vi "Traverse.vi"() -> ()   [LabVIEW 2011]
uses:
  Anemometry/Anemometry Sub Vis/Controls/User_Specific_mode.ctl
  Anemometry/Anemometry Sub Vis/Controls/Tunnel_Coordinates.ctl
  Anemometry/Anemometry Sub Vis/Gen Trav/Trav_mode.ctl
  <vilib>/Utility/file.llb/Write To Spreadsheet File (DBL).vi
panel:
  in  "Loop Delay (s)":u32=15
  in  "Minimum Depth into soution (mm)":dbl=1120.0
  in  "Number of Points Between Minimum and Maximum Depth":dbl=20.0
  in  "Maximum Depth into solution (mm)":dbl=1399.0
  in  "Save Location":path=path "C:/Documents and Settings/Adetola Elias/My Documents/Danial/Traverse Run Actual.xls"
  in  "Sample Size for Density Meter Reading":i32=20
  in  "Delay For Density Meter Reading (s)":u32=15
  # "Time from Traverse to Density Meter = 14 Sec"
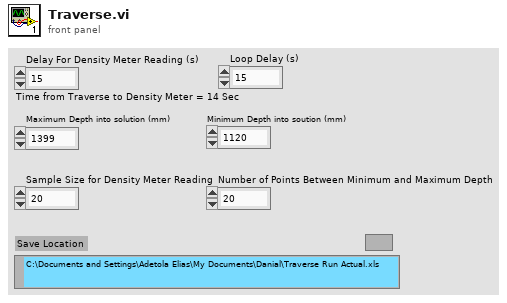
[diagram p1: front panel]
types:
  T1 = typedef "User_Specific_mode.ctl" = enum16{"Check VI only", "Run VI"}
  T2 = typedef "Tunnel_Coordinates.ctl" = enum16{"Work in Tunnel Coordinates", "Work in Model Coordinates"}
  T3 = typedef "Trav_mode.ctl" = enum16{"Move traverse", "Read traverse position", "Teach Position"}
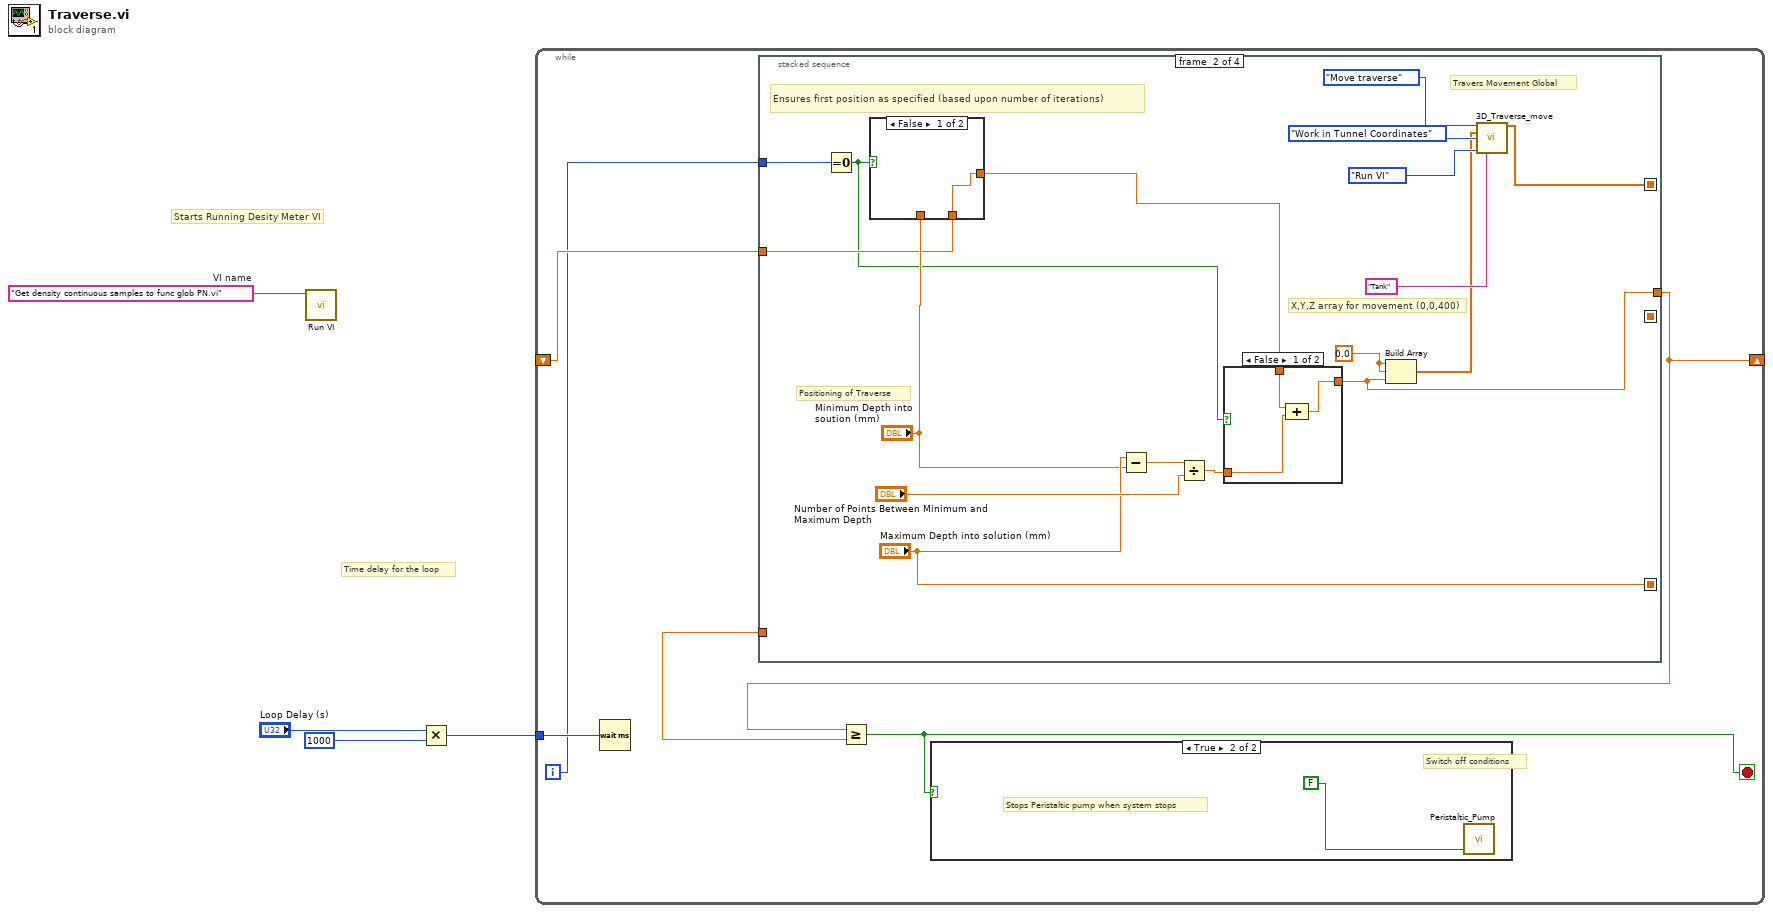
[diagram p0: block diagram]
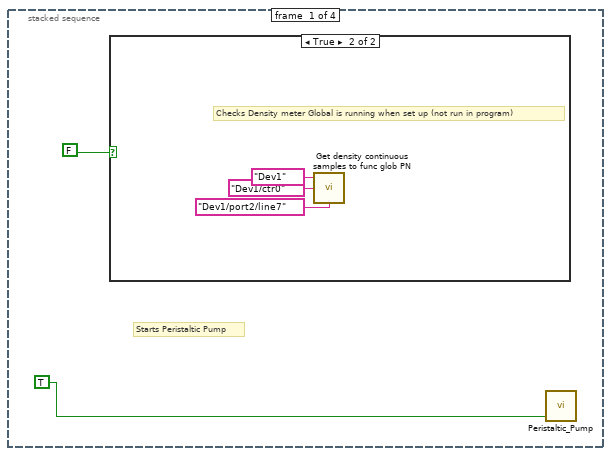
[diagram p3: hidden frame]
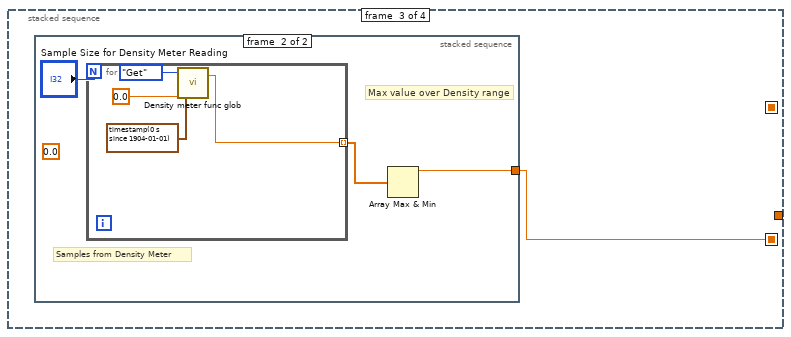
[diagram p7: hidden frame]
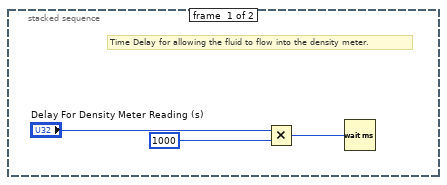
[diagram p8: hidden frame]
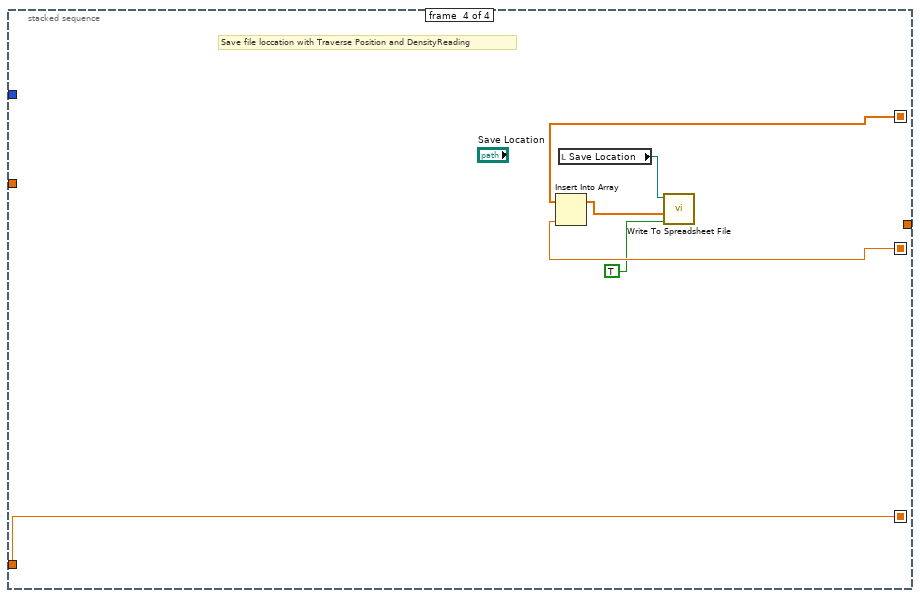
[diagram p9: hidden frame]
diagram:
  w3 = "Get density continuous samples to func glob PN.vi"  # VI name
  # "Time delay for the loop"
  # "Starts Running Desity Meter VI"
  n1 = call "Run VI.vi"("VI name"=w3) -> ()  [unwired: 11 in]
  n2 = Multiply(x="Loop Delay (s)", y=1000 ("Sample Size 2")) -> (x*y=w4:u32)
  n3 = while {
    tunnel: w4 -> [w9]
    shift-right: [w8] -> _
    shift-left: _ -> [w7]
    i -> [w5]
    stop <- w6 stop-if-true
    # "Switch off conditions"
    n4 = Wait (ms)(milliseconds to wait=w9) -> ()  [unwired: 1 out]
    n5 = stacked-sequence {
      seq-local: [_ _ w40 _] -> [_ _ _ w54]
      seq-local: [_ w26 _ _] -> [_ _ _ w53]
      seq-local: [_ "Maximum Depth into solution (mm)" _ _] -> [_ _ _ w52]
      tunnel: w7 -> [_ w18 _ _]
      tunnel: [_ w27 _ _] -> w8
      tunnel: [_ _ _ w52] -> w10
      tunnel: w5 -> [_ w21 _ _]
      frame #0 {
        # "Starts Peristaltic Pump"
        n6 = case shown="True" FALSE {
          frame False {
          }
          frame True {
            # "Checks Density meter Global is running when set up (not run in program)"
            n7 = call "Get density continuous samples to func glob PN.vi"("Timing SW trigger"=tag "Dev1/port2/line7", "Counter"=tag "Dev1/ctr0", "Device"=tag "Dev1") -> ()
          }
        }
        n8 = call "Peristaltic_Pump.vi"("Set state:"=TRUE) -> ()  [unwired: 3 in, 2 out]
      }
      frame #1 {
        w28 = 0.0 ("Density in")
        # "Positioning of Traverse"
        # "X,Y,Z array for movement (0,0,400)"
        # "Travers Movement Global"
        # "Ensures first position as specified (based upon number of iterations)"
        n9 = Equal To 0?(x=w21) -> (x = 0?=w17:bool)
        n10 = case shown="False" w17 {
          tunnel: [w34 w35] -> w19
          tunnel: "Minimum Depth into soution (mm)" -> [_ w35]
          tunnel: w18 -> [w34 _]
          frame False {
          }
          frame True {
          }
        }
        n11 = Subtract(x="Maximum Depth into solution (mm)", y="Minimum Depth into soution (mm)") -> (x-y=w25:dbl)
        n12 = Divide(x=w25, y="Number of Points Between Minimum and Maximum Depth") -> (x/y=w23:dbl)
        n13 = case shown="False" w17 {
          tunnel: w19 -> [w38 w39]
          tunnel: [w37 w39] -> w27
          tunnel: w23 -> [w36 _]
          frame False {
            n14 = Compound Arithmetic op=ADD(w38, w36) -> (w37:dbl)
          }
          frame True {
          }
        }
        n15 = Build Array(w28, w28, w27) -> (w29:dbl[])
        n16 = call "3D_Traverse_move.vi"("Mode"=Trav_mode."Move traverse", "Position"=w29, "Work in Tunnel Coordinates"=Tunnel_Coordinates."Work in Tunnel Coordinates", "Simulate/Run"=User_Specific_mode."Run VI", "Traverse name"="Tank") -> ("Trav Position achieved"=w26:dbl[])  [unwired: 8 in, 2 out]
      }
      frame #2 {
        n17 = stacked-sequence {
          tunnel: [_ w45] -> w40
          frame #0 {
            # "Time Delay for allowing the fluid to flow into the density meter."
            n18 = Multiply(x="Delay For Density Meter Reading (s)", y=1000 ("Sample Size 2")) -> (x*y=w42:u32)
            n19 = Wait (ms)(milliseconds to wait=w42) -> ()  [unwired: 1 out]
          }
          frame #1 {
            (unwired) 0.0 ("Actual Density (kg/m3) 2")
            # "Max value over Density range"
            # "Samples from Density Meter"
            n20 = for {
              N: "Sample Size for Density Meter Reading" -> [_]
              tunnel: [w47] -> w44 mode=indexing
              n21 = call "Density meter func glob.vi"("Sample DateTime in"=timestamp(0 s since 1904-01-01), "Density in"=0.0, "Action"=enum16{"Get", "Set"}."Get") -> ("Density out"=w47:dbl)  [unwired: 1 out]
            }
            n22 = Array Max & Min(array=w44) -> (max value=w45:dbl)  [unwired: 3 out]
          }
        }
      }
      frame #3 {
        # "Save file loccation with Traverse Position and DensityReading"
        n23 = Insert Into Array(array=w53, new element=w54) -> (w55:dbl[])  [unwired: 1 in]
        n24 = local read "Save Location"() -> (w56:path)
        n25 = call-poly <vilib>:"Write To Spreadsheet File.vi"("append to file? (new file:F)"=TRUE, "1D data"=w55, "file path (dialog if empty)"=w56) -> ()  [unwired: 5 in, 1 out]
      }
    }
    n26 = Greater Or Equal?(x=w8, y=w10) -> (x >= y?=w6:bool)
    n27 = case shown="True" w6 {
      frame False {
      }
      frame True {
        # "Stops Peristaltic pump when system stops"
        n28 = call "Peristaltic_Pump.vi"("Set state:"=FALSE) -> ()  [unwired: 3 in, 2 out]
      }
    }
  }
